vi "Test Delete All.vi"(8 "error in (no error)":errorcluster, 11 "Connection Refnum":T1) -> (0 "error out":errorcluster, 3 "Connection Refnum":T1)   [LabVIEW 2011]
uses:
  SI.LIB/ODBC/SQL Controls/Connection Refnum.ctl
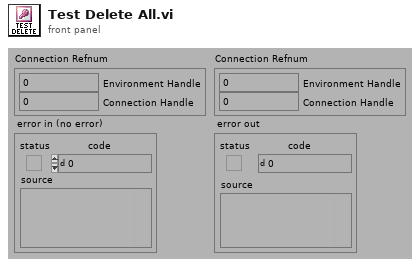
[diagram p1: front panel]
types:
  T1 = typedef "Connection Refnum.ctl" = cluster{"Environment Handle":i32, "Connection Handle":i32}
  T2 = typedef "Test Record.ctl" = cluster{"ixTest":i32, "sxTestId":string, "sVersion":string, "sDriverTypes":string[], "sDescription":string, "iQuickMode":i32}
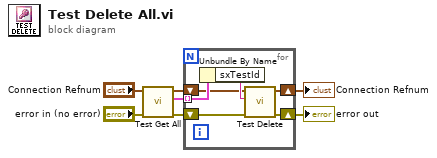
[diagram p0: block diagram]
diagram:
  n1 = call "Test Get All.vi"("error in (no error)"="error in (no error)", "Connection Refnum"="Connection Refnum") -> ("error out"=w7:errorcluster, "Test Records"=w6:T2[], "Connection Refnum"=w4:T1)  [unwired: 2 in, 5 out]
  n2 = for {
    shift-right: [w13] -> w1
    shift-left: w7 -> [w12]
    tunnel: w6 -> [w11] mode=indexing
    shift-right: [w8] -> w3
    shift-left: w4 -> [w9]
    n3 = Unbundle By Name(w11) -> ("sxTestId"=w10:string)
    n4 = call "Test Delete.vi"("error in (no error)"=w12, "sxTestId (\"\")"=w10, "Connection Refnum"=w9) -> ("error out"=w13:errorcluster, "Connection Refnum"=w8:T1)  [unwired: 7 out]
  }
  "error out" <- w1
  "Connection Refnum" <- w3
